vi "BonOMM-SAOMM.vi"() -> ()   [LabVIEW 2019] (continued)
                n727 = local read "XReference"() -> (w1202:dbl)
                n728 = local read "YReference"() -> (w1201:dbl)
                n729 = Greater?(x=w1207, y=w1208) -> (0:w1206:bool)
                n730 = expression code="x/180.0"(3.141592653589793) -> (w1195:dbl)
                n731 = call "xy2ad.vi"("Y (px)"=w1201, "X (px)"=w1202, "Astrometry"=w1203) -> ("DEC (°)"=w1198:dbl, "RA (°)"=w1199:dbl)  [unwired: 5 in, 2 out]
                n732 = call "xy2ad.vi"("Y (px)"=w1204, "X (px)"=w1205, "Astrometry"=w1203) -> ("DEC (°)"=w1196:dbl, "RA (°)"=w1197:dbl)  [unwired: 5 in, 2 out]
                n733 = case shown="Vrai" w1206 {
                  tunnel: w1207 -> [_ w1209]
                  frame False {
                  }
                  frame True {
                    "CorrID" <- w1209
                  }
                }
                n734 = formula code="ErrorRA=(CenRA-RefRA)*3600.0*cos(RefDEC*PIsur180);\nErrorDEC=(CenDEC-RefDEC)*3600.0;"("RefRA"=w1199, "RefDEC"=w1198, "CenRA"=w1197, "CenDEC"=w1196, "PIsur180"=w1195) -> ("ErrorRA"=w1194:dbl, "ErrorDEC"=w1193:dbl)
              }
              frame 2 {
                # "Ajouter une condition sur la dérivée locale ???"
                # "Asservissement Actif (LUT + Servo + Guidage)"
                # "Pas besoin d'appliquer la rotation puisque\nseul l'écart de l'hexapode est considéré."
                n735 = local read "EcartX"() -> (w1219:dbl)
                n736 = local read "EcartY"() -> (w1222:dbl)
                n737 = Absolute Value(x=w1219) -> (abs(x)=w1224:dbl)
                n738 = Absolute Value(x=w1222) -> (abs(x)=w1223:dbl)
                n739 = Greater Or Equal?(x=w1224, y="CorrTreshold") -> (x >= y?=w1218:bool)
                n740 = Less?(x="CorrTreshold", y=w1223) -> (x < y?=w1211:bool)
                n741 = Or(x=w1218, y=w1211) -> (x .or. y?=w1225:bool)
                n742 = Multiply(x=w1219, y="HexXRate") -> (x*y=w1217:dbl)
                n743 = Multiply(x="HexYRate", y=w1222) -> (x*y=w1214:dbl)
                n744 = Select(t=w1214, s=w1211, f=0.0) -> (s? t:f=w1213:dbl)
                n745 = Select(t=w1217, s=w1218, f=0.0) -> (s? t:f=w1215:dbl)
              }
              frame 4 {
                # "On  envoi la commande recu"
                # "Mode Guidage externe"
                n746 = local read "GE_TCS_DEC"() -> (w1232:dbl)
                n747 = local read "GE_TCS_RA"() -> (w1233:dbl)
                n748 = Not Equal To 0?(x=w1232) -> (x != 0?=w1229:bool)
                n749 = local read "GE_TCS"() -> (w1228:bool)
                n750 = Not Equal To 0?(x=w1233) -> (x != 0?=w1230:bool)
                n751 = Or(x=w1230, y=w1229) -> (x .or. y?=w1227:bool)
                n752 = And(x=w1227, y=w1228) -> (x .and. y?=w1231:bool)
                n753 = case shown="Vrai" w1231 {
                  frame False {
                  }
                  frame True {
                    # "On efface la commande"
                    n754 = local read "GE_TCS_DEC"() -> (w1234:dbl)
                    n755 = local read "GE_TCS_RA"() -> (w1240:dbl)
                    n756 = In Range and Coerce(upper limit=5.0, x=w1240, lower limit=-5.0) -> (In Range?=w1243:bool)  [unwired: 1 out]
                    n757 = In Range and Coerce(upper limit=5.0, x=w1234, lower limit=-5.0) -> (In Range?=w1235:bool)  [unwired: 1 out]
                    n758 = case shown="Faux" w1243 {
                      tunnel: w1240 -> [w1252 _]
                      tunnel: [w1253 0.0 ("GE_TCS_RA")] -> w1239
                      frame False {
                        n759 = Greater Than 0?(x=w1252) -> (x > 0?=w1254:bool)
                        n760 = case shown="Faux" w1254 {
                          tunnel: [-5.0 ("y") 5.0 ("y")] -> w1251
                          frame False {
                          }
                          frame True {
                          }
                        }
                        n761 = Subtract(x=w1252, y=w1251) -> (x-y=w1253:dbl)
                      }
                      frame True {
                      }
                    }
                    n762 = case shown="Faux" w1235 {
                      tunnel: [w1247 0.0 ("GE_TCS_DEC")] -> w1238
                      tunnel: w1234 -> [w1246 _]
                      frame False {
                        n763 = Greater Than 0?(x=w1246) -> (x > 0?=w1245:bool)
                        n764 = case shown="Faux" w1245 {
                          tunnel: [-5.0 ("y") 5.0 ("y")] -> w1244
                          frame False {
                          }
                          frame True {
                          }
                        }
                        n765 = Subtract(x=w1246, y=w1244) -> (x-y=w1247:dbl)
                      }
                      frame True {
                      }
                    }
                    n766 = local write "GE_TCS_RA"(w1239) -> ()
                    n767 = local write "GE_TCS_DEC"(w1238) -> ()
                  }
                }
              }
            }
            n768 = Tick Count (ms)() -> (millisecond timer value=w1179:u32)
            n769 = Subtract(x=w1179, y="LastCorr") -> (x-y=w1181:u32)
            n770 = Greater?(x=w1181, y="CorrDelay") -> (0:w1183:bool)
            n771 = local read "SNRtreshold"() -> (w1175:dbl)
            n772 = local read "SNR"() -> (w1176:dbl)
            n773 = local read "Servo"() -> (w1172:bool)
            n774 = Greater Or Equal?(x=w1176, y=w1175) -> (x >= y?=w1173:bool)
            n775 = Compound Arithmetic op=AND(w1173, w1172) -> (w1171:bool)
            n776 = Or(x=w1170, y=w1171) -> (x .or. y?=w1169:bool)
            n777 = Compound Arithmetic op=AND(w1177, w1169, w1183) -> (w1174:bool)
            n778 = case shown="Vrai" w1174 {
              tunnel: w1185 -> [_ w1293]
              tunnel: w1184 -> [_ w1292]
              tunnel: "Corr%" -> [_ w1294]
              frame False {
              }
              frame True {
                w1260 = -5000.0 ("lower limit")
                w1261 = 5000.0 ("x")
                # "millisecond d'activation\ndes relais ..."
                # "À déterminer sur l'ordinateur de BonOMM à OMM\nIl faut refaire le lien quand c'est sur un nouvel ordi"
                n779 = Tick Count (ms)() -> (millisecond timer value=w1296:u32)
                n780 = formula code="EW=(agg/100)*corrX*rRA;\nNS=(agg/100)*corrY*rDEC;"("agg"=w1294, "rRA"="RateRA", "bRA"="BacklashRA", "rDEC"="RateDEC", "bDEC"="BacklashDEC", "corrX"=w1292, "corrY"=w1293) -> ("NS"=w1291:dbl, "EW"=w1290:dbl)
                n781 = local write "LastCorr"(w1296) -> ()
                n782 = local read "path_trackfile"() -> (w1279:path)
                n783 = control-ref of="GuidingCancel"() -> (w1283:refnum<vi>)
                n784 = control-ref of="GuideNorth"() -> (w1284:refnum<vi>)
                n785 = control-ref of="GuideSouth"() -> (w1285:refnum<vi>)
                n786 = control-ref of="GuideEast"() -> (w1282:refnum<vi>)
                n787 = control-ref of="GuideWest"() -> (w1281:refnum<vi>)
                n788 = Round To Nearest(number=w1291) -> (nearest integer value=w1263:dbl)
                n789 = Round To Nearest(number=w1290) -> (nearest integer value=w1262:dbl)
                n790 = Strip Path(path=w1279) -> (stripped path=w1277:path)  [unwired: 1 out]
                n791 = In Range and Coerce(upper limit=w1261, x=w1263, lower limit=w1260) -> (coerced(x)=w1258:dbl)  [unwired: 1 out]
                n792 = In Range and Coerce(upper limit=w1261, x=w1262, lower limit=w1260) -> (coerced(x)=w1259:dbl)  [unwired: 1 out]
                n793 = Bundle("GuidingCancel"=w1283, "GuideNorth"=w1284, "GuideSouth"=w1285, "GuideEast"=w1282, "GuideWest"=w1281) -> (w1280:T27)  [unwired: 1 in]
                n794 = Build Path(base path=w1277, name or relative path="Relays") -> (appended path=w1264:path)
                n795 = local read "RotationTCS"() -> (w1272:dbl)
                n796 = local read "ErrX"() -> (w1270:string)
                n797 = local read "ErrY"() -> (w1269:string)
                n798 = local read "exptime"() -> (w1271:dbl)
                n799 = To Long Integer(number=w1258) -> (32bit integer=w1273:i32)
                n800 = To Long Integer(number=w1259) -> (32bit integer=w1274:i32)
                n801 = Fract/Exp String To Number(string=w1270) -> (number=w1268:dbl)  [unwired: 3 in, 1 out]
                n802 = Fract/Exp String To Number(string=w1269) -> (number=w1267:dbl)  [unwired: 3 in, 1 out]
                n803 = local read "HexX"() -> (w1266:dbl)
                n804 = local read "HexY"() -> (w1265:dbl)
                n805 = call "LogRelayData.vi"("Path"=w1264, "XCorr"=w1273, "YCorr"=w1274, "Rotation"=w1272, "Texp"=w1271, "CenX"=w1268, "CenY"=w1267, "XHex"=w1266, "YHex"=w1265) -> ()  [unwired: 7 in]
                n806 = call "DIO-ApplyCorrection.vi"("TaskCluster"=T21 {"North Task"="Nord", "West Task"="Sud", "South Task"="Est", "East Task"="Ouest"}, "NordSud(ms)"=w1273, "EstOuest(ms)"=w1274, "ReferenceCluster"=w1280) -> ("GuiderRA Error"=w1276:errorcluster, "GuiderDEC Error"=w1275:errorcluster)  [unwired: 10 in]
                n807 = call "LogRelayError.vi"("Path"=w1264, "GuiderRA Error"=w1276, "GuiderDEC Error"=w1275) -> ()  [unwired: 13 in]
              }
            }
            n808 = local read "Quit"() -> (w1178:bool)
            n809 = Wait Until Next ms Multiple(millisecond multiple=u32 50) -> ()  [unwired: 1 out]
          }
          "Guidage" <- w977
          n810 = while {
            tunnel: ["Quit"] -> w982
            stop <- "Quit" stop-if-true
            # "Structure de gestion des événements utilisateurs"
            n811 = event shown="[64] \"BoutonTest\": Valeur changée" {
              selector: _ -> [_ _ _ _ _ _ _ _ _ _ _ _ _ _ _ _ _ _ _ _ _ _ _ _ _ _ _ _ _ _ _ _ _ _ _ _ _ _ _ _ _ _ _ _ _ _ _ _ _ _ _ _ _ _ _ _ _ _ _ _ _ _ _ _ _ _ _ _]
              dyn-events: _ -> [_ _ _ _ _ _ _ _ _ _ _ _ _ _ _ _ _ _ _ _ _ _ _ _ _ _ _ _ _ _ _ _ _ _ _ _ _ _ _ _ _ _ _ _ _ _ _ _ _ _ _ _ _ _ _ _ _ _ _ _ _ _ _ _ _ _ _ _]
              timeout: 250 -> [_ _ _ _ _ _ _ _ _ _ _ _ _ _ _ _ _ _ _ _ _ _ _ _ _ _ _ _ _ _ _ _ _ _ _ _ _ _ _ _ _ _ _ _ _ _ _ _ _ _ _ _ _ _ _ _ _ _ _ _ _ _ _ _ _ _ _ _]
              event Timeout {
                w4204 = FALSE
                # "S'il y a un problème avec MC-BonOMM, regarder ici ;)"
                # "Test pour les boutons de Jog ..."
                n812 = event-data() -> ()  [unwired: 1 in, 1 out]
                n813 = local write "Annulation en cours"(FALSE) -> ()
                n814 = disable-structure shown="Enabled" {
                  frame Disabled {
                    n815 = local read "MC-BonOMM VRN"() -> (w4206:refnum<visa-resource-name>)
                    n816 = property class="Instr"(reference=w4206) -> (reference out=w4207:refnum<visa-resource-name>, "Serial Settings:Number of Bytes at Serial Port"=w4208:u32)  [unwired: 1 in, 1 out]
                    n817 = VISA Read(VISA resource name=w4207, byte count=w4208) -> ()  [unwired: 1 in, 4 out]
                  }
                  frame Enabled {
                  }
                }
                n818 = local write "go Nord"(w4204) -> ()
                n819 = local write "go Ouest"(w4204) -> ()
                n820 = local write "go Est"(w4204) -> ()
                n821 = local write "go Sud"(w4204) -> ()
                n822 = local write "enfoncé"(w4204) -> ()
              }
              event Menu Selection (User) {
                n823 = event-data() -> ("MenuRef"=w4209:refnum<k9>, "ItemTag"=w4211:string, "ItemPath"=w4212:string)  [unwired: 1 in, 3 out]
                n824 = Concatenate Strings(":" ("search string/char (-)"), w4211) -> (w4213:string)
                n825 = Search/Split String(string=w4212, search string/char (-)=w4213) -> (substring before match=w4210:string)  [unwired: 1 in, 2 out]
                n826 = case shown="\"main_Secondaire Actif\"" w4210 {
                  tunnel: w4211 -> [_ w4215 w4532 w4563 w4693 w4768 w4862 w4956 w5019 w5044]
                  tunnel: w4209 -> [_ _ _ _ _ _ w4861 _ _ _]
                  frame Default {
                  }
                  frame "main_Communications" {
                    # "Gestion des éléments du menu \"communications\"\n(fermeture de la connexion, puis redémarrage)"
                    n827 = case shown="\"com_Telescope Control System\"" w4215 {
                      frame Default {
                        (unwired) FALSE ("Boolean")
                      }
                      frame "com_Telescope Control System" {
                        n828 = flat-sequence {
                          frame #0 {
                            w4229 = "communications" ("name or relative path")
                            n829 = control-ref of="TCS actif"() -> (w4218:refnum<vi>)
                            n830 = local read "TCS VRN"() -> (w4223:refnum<visa-resource-name>)
                            n831 = call "EXCOM-25-EQ.vi"("VISA resource name"=w4223, "Bool Refnum"=w4218) -> ("VISA resource name dup"=w4221:refnum<visa-resource-name>, "Error OUT"=w4222:errorcluster)  [unwired: 3 in, 13 out]
                            n832 = local read "properties.ini"() -> (w4225:path)
                            n833 = call "SerialCommError.vi"("VISA IN"=w4221, "error IN"=w4222) -> ("VISA OUT"=w4236:refnum<visa-resource-name>, "Error"=w4224:bool, "error OUT"=w4216:errorcluster)  [unwired: 11 in]
                            n834 = Not(x=w4224) -> (.not. x?=w4217:bool)
                            n835 = call <vilib>:"Open Config Data.vi"("configuration file path"=w4225) -> ("error out"=w4234:errorcluster, "refnum"=w4235:T23)  [unwired: 8 in, 1 out]
                            n836 = local write "TCS VRN"(w4236) -> ()
                            n837 = local write "TCS Error"(w4216) -> ()
                            n838 = case shown="Vrai" w4217 {
                              tunnel: [TRUE ("Boolean") w4279] -> w4219
                              frame False {
                              }
                              frame True {
                                n839 = Two Button Dialog(message="La connexion TCP/IP semble fonctionner.\nDésirez-vous vraiment la réinitialiser ?" ("T button name (\"OK\")"), 1:"Non" ("F button name (\"Cancel\")"), 2:"Oui" ("T button name (\"OK\")")) -> (T button?=w4279:bool)
                              }
                            }
                            n840 = call-poly <vilib>:"Read Key.vi"("section"=w4229, "error in (no error)"=w4234, "key"="TCS-IP" ("name or relative path"), "refnum"=w4235) -> ("error out"=w4232:errorcluster, "value"=w4220:string, "refnum out"=w4233:T23)  [unwired: 4 in, 1 out]
                            n841 = call-poly <vilib>:"Read Key.vi"("section"=w4229, "error in (no error)"=w4232, "key"="TCS-PN" ("name or relative path"), "refnum"=w4233) -> ("error out"=w4230:errorcluster, "value"=w4226:u32, "refnum out"=w4231:T23)  [unwired: 4 in, 1 out]
                            n842 = call <vilib>:"Close Config Data.vi"("error in (no error)"=w4230, "refnum"=w4231) -> ()  [unwired: 8 in, 2 out]
                            n843 = case shown="Vrai" w4219 {
                              tunnel: w4226 -> [_ w4242]
                              tunnel: w4220 -> [_ w4243]
                              tunnel: w4218 -> [_ w4244]
                              frame False {
                              }
                              frame True {
                                n844 = flat-sequence {
                                tunnel: w4244 -> [w4251]
                                tunnel: [refnum<visa-resource-name> "-1" ("Table VRN")] -> w4239
                                tunnel: [w4248] -> w4238
                                tunnel: w4239 -> [w4255]
                                tunnel: w4238 -> [w4254]
                                tunnel: [w4252] -> w4237
                                tunnel: w4237 -> [_]
                                tunnel: w4243 -> [w4262]
                                tunnel: w4242 -> [w4261]
                                tunnel: [w4260] -> w4241
                                tunnel: [w4259] -> w4240
                                tunnel: [w4273] -> w4246
                                tunnel: [w4272] -> w4245
                                tunnel: w4240 -> [_]
                                tunnel: w4241 -> [w4267]
                                tunnel: w4246 -> [w4275]
                                tunnel: w4245 -> [w4274]
                                frame #0 {
                                w4247 = TRUE ("TCS R actif")
                                n845 = local write "ReconnectionMute"(w4247) -> ()
                                n846 = local read "TCS VRN"() -> (w4248:refnum<visa-resource-name>)
                                n847 = call "TCS-Wait4Flag.vi"("Raise Flag ?"=TRUE, "Ctl Refnum IN"=w4251) -> ()  [unwired: 8 in, 2 out]
                                "TCSMute" <- w4247
                                }
                                frame #1 {
                                n848 = local write "TCS VRN"(w4255) -> ()
                                n849 = Type Cast(type=refnum<k5> refnum ("connection ID out"), x=w4254) -> (*(type *) &x=w4256:refnum<k5>)
                                n850 = TCP Close Connection(connection ID=w4256) -> (error out=w4252:errorcluster)  [unwired: 2 in, 1 out]
                                }
                                frame #2 {
                                n851 = Wait (ms)(milliseconds to wait=u32 1000) -> ()  [unwired: 1 out]
                                }
                                frame #3 {
                                n852 = To Unsigned Word Integer(number=w4261) -> (unsigned 16bit integer=w4263:u16)
                                n853 = local write "TCS actif"(FALSE ("TCS R actif")) -> ()
                                n854 = TCP Open Connection(address=w4262, remote port or service name=w4263) -> (connection ID=w4260:refnum<k5>, error out=w4259:errorcluster)  [unwired: 3 in]
                                }
                                frame #4 {
                                # "Doit-on fermer la \nconnexion d'abord ?"
                                n855 = Type Cast(type="", x=w4267) -> (*(type *) &x=w4270:string)
                                n856 = control-ref of="TCS actif"() -> (w4264:refnum<vi>)
                                n857 = Type Cast(type=refnum<visa-resource-name> "-1" ("Table VRN"), x=w4270) -> (*(type *) &x=w4268:refnum<visa-resource-name>)
                                n858 = call "EXCOM-25-EQ.vi"("VISA resource name"=w4268, "Bool Refnum"=w4264) -> ("VISA resource name dup"=w4266:refnum<visa-resource-name>, "Error OUT"=w4265:errorcluster)  [unwired: 3 in, 13 out]
                                n859 = call "SerialCommError.vi"("VISA IN"=w4266, "error IN"=w4265) -> ("VISA OUT"=w4273:refnum<visa-resource-name>, "error OUT"=w4272:errorcluster)  [unwired: 11 in, 1 out]
                                }
                                frame #5 {
                                n860 = case shown="Erreur" w4274 {
                                frame No Error {
                                }
                                frame Error {
                                n861 = One Button Dialog(message="La communication avec le TCS ne semble toujours pas foncitonner.\nVérifiez les connexions et les paramètres puis recommencez." ("T button name (\"OK\")")) -> ()  [unwired: 1 in, 1 out]
                                }
                                }
                                n862 = local write "TCS Error"(w4274) -> ()
                                n863 = local write "TCS VRN"(w4275) -> ()
                                }
                                frame #6 {
                                w4277 = FALSE
                                n864 = local write "ReconnectionMute"(w4277) -> ()
                                n865 = local write "TCSMute"(w4277) -> ()
                                }
                                }
                              }
                            }
                          }
                        }
                      }
                      frame "com_Caméra de référence" {
                        n866 = local read "exptime"() -> (w4285:dbl)
                        n867 = local read "MessageType"() -> (w4290:cluster{string[], u32[]})
                        n868 = control-ref of="PrAMS-ACK"() -> (w4295:refnum<vi>)
                        n869 = control-ref of="PrAMS actif"() -> (w4294:refnum<vi>)
                        n870 = local read "Signature"() -> (w4293:u32)
                        n871 = local read "PrAMS VRN"() -> (w4296:refnum<visa-resource-name>)
                        n872 = expression code="x*1000"(w4285) -> (w4288:dbl)
                        n873 = To Unsigned Long Integer(number=w4288) -> (unsigned 32bit integer=w4287:u32)
                        n874 = call-poly "SAOMM-Num2littleEndian.vi"("Number"=w4287) -> ("LiitleEndianedData"=w4286:u8[])  [unwired: 14 in]
                        n875 = call "SAOMM-SendSET.vi"("PRAMMS-COMM IN"=w4296, "Active Refnum"=w4294, "PrAMS-ACK"=w4295, "Signature"=w4293, "Error IN"=errorcluster {"status"=FALSE, "code"=0, "source"=""} ("PRAMMS Error"), "MessageType"=w4290, "Active SET"="emtSetImageExposureTime", "Value (little endianed byte array)"=w4286) -> ("Error"=w4284:bool, "Error OUT"=w4292:errorcluster)  [unwired: 4 in, 2 out]
                        n876 = local write "PrAMS Error"(w4292) -> ()
                        n877 = Not(x=w4284) -> (.not. x?=w4283:bool)
                        n878 = case shown="Vrai" w4283 {
                          tunnel: [TRUE ("Boolean") w4299] -> w4297
                          frame False {
                          }
                          frame True {
                            n879 = Two Button Dialog(message="La connexion TCP/IP semble fonctionner.\nDésirez-vous vraiment la réinitialiser ?" ("T button name (\"OK\")"), 1:"Non" ("F button name (\"Cancel\")"), 2:"Oui" ("T button name (\"OK\")")) -> (T button?=w4299:bool)
                          }
                        }
                        n880 = case shown="Vrai" w4297 {
                          frame False {
                          }
                          frame True {
                            n881 = flat-sequence {
                              tunnel: [w4304] -> w4303
                              tunnel: w4303 -> [_]
                              frame #0 {
                                n882 = local read "PrAMS VRN"() -> (w4306:refnum<visa-resource-name>)
                                n883 = Type Cast(type=refnum<k5> refnum ("connection ID"), x=w4306) -> (*(type *) &x=w4305:refnum<k5>)
                                n884 = TCP Close Connection(connection ID=w4305) -> (error out=w4304:errorcluster)  [unwired: 2 in, 1 out]
                              }
                              frame #1 {
                                n885 = local read "properties.ini"() -> (w4316:path)
                                n886 = local read "path_config"() -> (w4309:path)
                                n887 = Build Path(base path=w4309, name or relative path=path "command.ini" ("command.ini")) -> (appended path=w4308:path)
                                n888 = call <vilib>:"Open Config Data.vi"("create file if necessary (T)"=FALSE, "configuration file path"=w4316) -> ("error out"=w4314:errorcluster, "refnum"=w4313:T23)  [unwired: 7 in, 1 out]
                                n889 = local read "Signature"() -> (w4325:u32)
                                n890 = call-poly <vilib>:"Read Key.vi"("section"="communications" ("key"), "error in (no error)"=w4314, "key"="PRAMMS-IP", "refnum"=w4313) -> ("error out"=w4320:errorcluster, "value"=w4312:string, "refnum out"=w4319:T23)  [unwired: 4 in, 1 out]
                                n891 = call <vilib>:"Close Config Data.vi"("error in (no error)"=w4320, "refnum"=w4319) -> ()  [unwired: 8 in, 2 out]
                                n892 = call "SAOMM-connect.vi"("IP"=w4312, "Port"=u16 10010, "Signature"=w4325, "Command.ini"=w4308) -> ("connection ID"=w4322:refnum<k5>, "Error OUT"=w4311:errorcluster)  [unwired: 7 in, 3 out]
                                n893 = disable-structure shown="Disabled" {
                                disable-tunnel: w4311 -> [w4327 _]
                                frame Disabled {
                                n894 = case shown="Erreur" w4327 {
                                frame No Error {
                                }
                                frame Error {
                                n895 = One Button Dialog(message="Erreur lors de la connexion\nà l'hexapode-console.") -> ()  [unwired: 1 in, 1 out]
                                }
                                }
                                }
                                frame Enabled {
                                }
                                }
                                n896 = local read "PrAMS VRN"() -> (w4324:refnum<visa-resource-name>)
                                n897 = local write "PrAMS Error"(w4311) -> ()
                                n898 = Type Cast(type=w4312, x=w4322) -> (*(type *) &x=w4321:string)
                                n899 = Type Cast(type=w4324, x=w4321) -> (*(type *) &x=w4323:refnum<visa-resource-name>)
                                n900 = local write "PrAMS VRN"(w4323) -> ()
                              }
                            }
                          }
                        }
                      }
                      frame "com_Tables de guidage" {
                        n901 = flat-sequence {
                          frame #0 {
                            w4330 = TRUE
                            n902 = local write "Sync_Ready"(FALSE ("Sync_Ready")) -> ()
                            "TableMute" <- w4330
                            "ReconnectionMute" <- w4330
                          }
                          frame #1 {
                            w4345 = "communications" ("name or relative path")
                            n903 = local read "Table VRN"() -> (w4334:refnum<visa-resource-name>)
                            n904 = local read "properties.ini"() -> (w4338:path)
                            n905 = control-ref of="Table actif"() -> (w4332:refnum<vi>)
                            n906 = local read "ActiveStages"() -> (w4331:string[])
                            n907 = call "Newmark-Status-All.vi"("Table VRN IN"=w4334, "Bool Refnum"=w4332, "StageTag"=w4331) -> ("Table VRN OUT"=w4335:refnum<visa-resource-name>, "Error OUT"=w4333:errorcluster)  [unwired: 4 in, 11 out]
                            n908 = call <vilib>:"Open Config Data.vi"("configuration file path"=w4338) -> ("error out"=w4350:errorcluster, "refnum"=w4351:T23)  [unwired: 8 in, 1 out]
                            n909 = call "SerialCommError.vi"("VISA IN"=w4335, "error IN"=w4333) -> ("VISA OUT"=w4352:refnum<visa-resource-name>, "Error"=w4336:bool)  [unwired: 11 in, 1 out]
                            n910 = case shown="Vrai" w4336 {
                              selector: w4336 -> [_ w4365]
                              tunnel: [w4361 w4365] -> w4337
                              frame False {
                                n911 = Two Button Dialog(message="La communication avec les tables semble bonne.\nDésirez-vous vraiment le réinitialiser ?" ("T button name (\"OK\")"), 1:"Non" ("F button name (\"Cancel\")"), 2:"Oui" ("T button name (\"OK\")")) -> (T button?=w4361:bool)
                              }
                              frame True {
                              }
                            }
                            n912 = call-poly <vilib>:"Read Key.vi"("section"=w4345, "error in (no error)"=w4350, "key"="tablevrn" ("name or relative path"), "refnum"=w4351) -> ("error out"=w4348:errorcluster, "value"=w4341:string, "refnum out"=w4349:T23)  [unwired: 4 in, 1 out]
                            n913 = local write "Table VRN"(w4352) -> ()
                            n914 = call-poly <vilib>:"Read Key.vi"("section"=w4345, "error in (no error)"=w4348, "key"="tablespd" ("name or relative path"), "refnum"=w4349) -> ("error out"=w4346:errorcluster, "value"=w4342:u32, "refnum out"=w4347:T23)  [unwired: 4 in, 1 out]
                            n915 = Type Cast(type=refnum<visa-resource-name> "-1" ("TCS R VRN"), x=w4341) -> (*(type *) &x=w4339:refnum<visa-resource-name>)
                            n916 = call <vilib>:"Close Config Data.vi"("error in (no error)"=w4346, "refnum"=w4347) -> ()  [unwired: 8 in, 2 out]
                            n917 = case shown="Vrai" w4337 {
                              tunnel: w4342 -> [_ w4358]
                              tunnel: w4339 -> [_ w4357]
                              frame False {
                              }
                              frame True {
                                n918 = local write "Table Baud rate"(w4358) -> ()
                                n919 = control-ref of="Table actif"() -> (w4355:refnum<vi>)
                                n920 = local read "ActiveStages"() -> (w4356:string[])
                                n921 = call "Newmark-Initialize.vi"("VISA resource name"=w4357, "ActiveStages"=w4356, "baud rate"=w4358, "Timeout"=u32 1000, "Bool Refnum"=w4355) -> ("VISA resource name out"=w4359:refnum<visa-resource-name>, "Error OUT"=w4353:errorcluster)  [unwired: 8 in, 1 out]
                                n922 = local write "Table Error"(w4353) -> ()
                                n923 = case shown="Pas d'erreur" w4353 {
                                frame No Error {
                                }
                                frame Error {
                                n924 = One Button Dialog(message="La communication avec les tables  ne semble toujours pas foncitonner.\nVérifiez les connexions et les paramètres puis recommencez." ("T button name (\"OK\")")) -> ()  [unwired: 1 in, 1 out]
                                }
                                }
                                n925 = local write "Table VRN"(w4359) -> ()
                              }
                            }
                          }
                          frame #2 {
                            w4367 = FALSE
                            n926 = local write "ReconnectionMute"(w4367) -> ()
                            n927 = local write "Sync_Ready"(TRUE ("Sync_Ready")) -> ()
                            n928 = local write "TableMute"(w4367) -> ()
                          }
                        }
                      }
                      frame "com_Secondaire Actif" {
                        (unwired) FALSE
                        w4377 = "communications" ("name or relative path")
                        n929 = local read "properties.ini"() -> (w4372:path)
                        n930 = call <vilib>:"Open Config Data.vi"("configuration file path"=w4372) -> ("error out"=w4382:errorcluster, "refnum"=w4383:T23)  [unwired: 8 in, 1 out]
                        n931 = One Button Dialog(message="À compléter ...") -> ()  [unwired: 1 in, 1 out]
                        n932 = call-poly <vilib>:"Read Key.vi"("section"=w4377, "error in (no error)"=w4382, "key"="PRAMMS-IP" ("name or relative path"), "refnum"=w4383) -> ("error out"=w4380:errorcluster, "value"=w4374:string, "refnum out"=w4381:T23)  [unwired: 4 in, 1 out]
                        n933 = call-poly <vilib>:"Read Key.vi"("section"=w4377, "error in (no error)"=w4380, "key"="PRAMMS-IP" ("name or relative path"), "refnum"=w4381) -> ("error out"=w4378:errorcluster, "value"=w4371:u32, "refnum out"=w4379:T23)  [unwired: 4 in, 1 out]
                        n934 = Type Cast(type=refnum<visa-resource-name> "-1" ("TCS R VRN"), x=w4374) -> (*(type *) &x=w4370:refnum<visa-resource-name>)
                        n935 = call <vilib>:"Close Config Data.vi"("error in (no error)"=w4378, "refnum"=w4379) -> ()  [unwired: 8 in, 2 out]
                        n936 = case shown="Vrai" TRUE {
                          tunnel: w4371 -> [_ _]
                          tunnel: w4370 -> [_ _]
                          frame False {
                          }
                          frame True {
                          }
                        }
                      }
                      frame "com_Lampes de calibration" {
                        n937 = flat-sequence {
                          frame #0 {
                            w4391 = "communications" ("name or relative path")
                            n938 = local read "properties.ini"() -> (w4384:path)
                            n939 = call <vilib>:"Open Config Data.vi"("configuration file path"=w4384) -> ("error out"=w4386:errorcluster, "refnum"=w4385:T23)  [unwired: 8 in, 1 out]
                            n940 = call-poly <vilib>:"Read Key.vi"("section"=w4391, "error in (no error)"=w4386, "key"="calibvrn" ("name or relative path"), "refnum"=w4385) -> ("error out"=w4388:errorcluster, "value"=w4394:string, "refnum out"=w4387:T23)  [unwired: 4 in, 1 out]
                            n941 = call-poly <vilib>:"Read Key.vi"("section"=w4391, "error in (no error)"=w4388, "key"="calibspd" ("name or relative path"), "refnum"=w4387) -> ("error out"=w4390:errorcluster, "value"=w4397:u32, "refnum out"=w4389:T23)  [unwired: 4 in, 1 out]
                            n942 = Type Cast(type=refnum<visa-resource-name> "-1" ("TCS R VRN"), x=w4394) -> (*(type *) &x=w4396:refnum<visa-resource-name>)
                            n943 = call <vilib>:"Close Config Data.vi"("error in (no error)"=w4390, "refnum"=w4389) -> ()  [unwired: 8 in, 2 out]
                            n944 = call-poly "VISA Configure Serial Port"("VISA resource name"=w4396, "timeout (10sec)"=u32 2000, "Enable Termination\nChar (T)"=FALSE ("Enable Termination\nChar (T)"), "baud rate (9600)"=w4397) -> ("VISA resource name out"=w4400:refnum<visa-resource-name>, "error out"=w4401:errorcluster)  [unwired: 10 in]
                            n945 = call "SerialCommError.vi"("VISA IN"=w4400, "error IN"=w4401) -> ("VISA OUT"=w4402:refnum<visa-resource-name>)  [unwired: 11 in, 2 out]
                            n946 = local write "Calib VRN"(w4402) -> ()
                          }
                          frame #1 {
                            n947 = One Button Dialog(message="Le port série des lampes de calibration a été réinitialisé.\n(Aucun test réel car la communication est à sens unique)") -> ()  [unwired: 1 in, 1 out]
                          }
                        }
                      }
                      frame "com_Commandes externes" {
                        (unwired) TRUE
                        n948 = flat-sequence {
                          frame #0 {
                            w4412 = "communications" ("name or relative path")
                            n949 = local read "properties.ini"() -> (w4405:path)
                            n950 = call <vilib>:"Open Config Data.vi"("configuration file path"=w4405) -> ("error out"=w4407:errorcluster, "refnum"=w4406:T23)  [unwired: 8 in, 1 out]
                            n951 = call-poly <vilib>:"Read Key.vi"("section"=w4412, "error in (no error)"=w4407, "key"="excvrn" ("name or relative path"), "refnum"=w4406) -> ("error out"=w4409:errorcluster, "value"=w4415:string, "refnum out"=w4408:T23)  [unwired: 4 in, 1 out]
                            n952 = call-poly <vilib>:"Read Key.vi"("section"=w4412, "error in (no error)"=w4409, "key"="excspd" ("name or relative path"), "refnum"=w4408) -> ("error out"=w4411:errorcluster, "value"=w4418:u32, "refnum out"=w4410:T23)  [unwired: 4 in, 1 out]
                            n953 = Type Cast(type=refnum<visa-resource-name> "-1" ("TCS R VRN"), x=w4415) -> (*(type *) &x=w4417:refnum<visa-resource-name>)
                            n954 = call <vilib>:"Close Config Data.vi"("error in (no error)"=w4411, "refnum"=w4410) -> ()  [unwired: 8 in, 2 out]
                            n955 = call-poly "VISA Configure Serial Port"("VISA resource name"=w4417, "timeout (10sec)"=u32 2000, "Enable Termination\nChar (T)"=FALSE ("Enable Termination\nChar (T)"), "baud rate (9600)"=w4418) -> ("VISA resource name out"=w4421:refnum<visa-resource-name>, "error out"=w4422:errorcluster)  [unwired: 10 in]
                            n956 = call "SerialCommError.vi"("VISA IN"=w4421, "error IN"=w4422) -> ("VISA OUT"=w4404:refnum<visa-resource-name>)  [unwired: 11 in, 2 out]
                            n957 = local write "Excmd VRN"(w4404) -> ()
                          }
                          frame #1 {
                            n958 = One Button Dialog(message="Le port série des communications externes a été réinitialisé.\n(Relancez une commande externe afin de tester la communication)") -> ()  [unwired: 1 in, 1 out]
                          }
                        }
                      }
                      frame "com_MC-BonOMM" {
                        n959 = local read "Périphérique"() -> (w4433:u16)
                        n960 = Two Button Dialog(message="Ceci va redémarrer le contrôleur de roue à filtre\net réinitialiser la communication.\nVoulez-vous continuer ?", 1:"NON" ("F button name (\"Cancel\")"), 2:"OUI" ("T button name (\"OK\")")) -> (T button?=w4424:bool)
                        n961 = Equal?(x=w4433, y=u16 0) -> (x = y?=w4435:bool)
                        n962 = Equal?(x=w4433, y=u16 1) -> (x = y?=w4434:bool)
                        n963 = Equal?(x=w4433, y=u16 2) -> (x = y?=w4436:bool)
                        n964 = Build Array(w4435, w4434, w4436) -> (w4428:bool[])
                        n965 = Boolean Array To Number(Boolean array=w4428) -> (number=w4429:u32)
                        n966 = case shown="Vrai" w4424 {
                          tunnel: w4429 -> [_ w4440]
                          tunnel: [w4437 w4438] -> _
                          frame False {
                            n967 = local read "MC_connect"() -> (w4437:bool)
                          }
                          frame True {
                            n968 = flat-sequence {
                              tunnel: w4440 -> [w4444]
                              tunnel: [w4444] -> w4439
                              tunnel: w4439 -> [w4464]
                              tunnel: [w4450] -> w4438
                              frame #0 {
                                n969 = local read "MC-BonOMM VRN"() -> (w4443:refnum<visa-resource-name>)
                                n970 = flat-sequence {
                                tunnel: w4441 -> [w4448]
                                frame #0 {
                                n971 = Wait (ms)(milliseconds to wait=u32 2000) -> ()  [unwired: 1 out]
                                }
                                frame #1 {
                                n972 = property class="Instr"(reference=w4448) -> (reference out=w4447:refnum<visa-resource-name>, "Serial Settings:Number of Bytes at Serial Port"=w4446:u32)  [unwired: 1 in, 1 out]
                                n973 = local write "MC_connect"(FALSE ("MC_connect")) -> ()
                                n974 = VISA Read(VISA resource name=w4447, byte count=w4446) -> ()  [unwired: 1 in, 4 out]
                                }
                                }
                                n975 = VISA Write(VISA resource name=w4443, write buffer="r" ("Commande")) -> (VISA resource name out=w4441:refnum<visa-resource-name>)  [unwired: 1 in, 2 out]
                              }
                              frame #1 {
                                n976 = local read "MC-BonOMM VRN"() -> (w4460:refnum<visa-resource-name>)
                                n977 = call "MC-BonOMM_talker.vi"("MC-BonOMM VRN"=w4460, "Commande"="m", "byte count"=u32 1, "Timeout (ms)"=2000, "answer=command?"=FALSE) -> ("Answer"=w4454:string, "ok ?"=w4457:bool)
                                n978 = Equal?(x="f", y=w4454) -> (x = y?=w4453:bool)
                                n979 = Equal?(x=w4454, y="x") -> (x = y?=w4452:bool)
                                n980 = Or(x=w4453, y=w4452) -> (x .or. y?=w4451:bool)
                                n981 = And(x=w4451, y=w4457) -> (x .and. y?=w4458:bool)
                                n982 = case shown="Vrai" w4458 {
                                tunnel: w4464 -> [_ w4470]
                                tunnel: [w4465 w4469] -> w4450
                                frame False {
                                n983 = One Button Dialog(message="Problème de communication avec MC-BonOMM", button name ("OK")="Oups :(") -> (true=w4466:bool)
                                n984 = Not(x=w4466) -> (.not. x?=w4465:bool)
                                }
                                frame True {
                                n985 = stacked-sequence {
                                tunnel: w4470 -> [w4472 w4483]
                                tunnel: [_ w4481] -> w4469
                                frame #0 {
                                n986 = case shown="1, Par défaut" w4472 {
                                tunnel: ["f" "o" "x"] -> w4471
                                frame 1, Default {
                                }
                                frame 2 {
                                }
                                frame 4 {
                                }
                                }
                                n987 = local read "MC-BonOMM VRN"() -> (w4475:refnum<visa-resource-name>)
                                n988 = call "MC-BonOMM_talker.vi"("MC-BonOMM VRN"=w4475, "Commande"=w4471, "Timeout (ms)"=2000, "answer=command?"=TRUE) -> ("ok ?"=w4473:bool)  [unwired: 1 in, 1 out]
                                n989 = case shown="Faux" w4473 {
                                frame False {
                                n990 = One Button Dialog(message="Erreur lors du changement de mode ...") -> ()  [unwired: 1 in, 1 out]
                                }
                                frame True {
                                }
                                }
                                n991 = local write "MC_connect"(w4473) -> ()
                                }
                                frame #1 {
                                n992 = local read "MC-BonOMM VRN"() -> (w4482:refnum<visa-resource-name>)
                                n993 = case shown="1, 2, Par défaut" w4483 {
                                tunnel: w4482 -> [w4489 w4499]
                                tunnel: [w4487 w4498] -> w4481
                                frame 1, 2, Default {
                                n994 = call "MC-BonOMM_talker.vi"("MC-BonOMM VRN"=w4489, "Commande"="q", "byte count"=u32 1, "Timeout (ms)"=8000, "answer=command?"=FALSE) -> ("Answer"=w4488:string, "ok ?"=w4487:bool)
                                n995 = Decimal String To Number(string=w4488) -> (number=w4492:i32)  [unwired: 2 in, 1 out]
                                n996 = local write "F#"(w4492) -> ()
                                n997 = case shown="1..6" w4492 {
                                selector: w4492 -> [w4494 _]
                                tunnel: [w4493 ""] -> w4491
                                frame 1..6 {
                                n998 = local read "Tableau des filtres"() -> (w4495:string[])
                                n999 = Decrement(x=w4494) -> (x-1=w4496:i32)
                                n1000 = Index Array(array=w4495, index=w4496) -> (element=w4493:string)
                                }
                                frame 0, Default {
                                }
                                }
                                n1001 = local write "filtre_nom"(w4491) -> ()
                                }
                                frame 4 {
                                n1002 = local read "ST_SPD"() -> (w4500:dbl)
                                n1003 = call "Change_speed.vi"("ST_SPD"=w4500, "MC-BonOMM VRN"=w4499) -> ("Connected?"=w4498:bool)
                                n1004 = case shown="Faux" w4498 {
                                frame False {
                                n1005 = property on="Périphérique" class="MDér (strict)"("Value (Signaling)"=u16 3) -> ()  [unwired: 2 in, 2 out]
                                }
                                frame True {
                                }
                                }
                                }
                                }
                                }
                                }
                                }
                                }
                                n1006 = local write "MC_connect"(w4450) -> ()
                              }
                            }
                          }
                        }
                      }
                      frame "com_Station Météo" {
                        # "Réinitialisation de la connexion avec le cRIO de météo"
                        n1007 = flat-sequence {
                          tunnel: [w4508] -> w4503
                          tunnel: w4503 -> [w4526]
                          tunnel: [w4526] -> w4502
                          frame #0 {
                            # "Ferme la connexion si elle est ouverte"
                            n1008 = local read "Cx"() -> (w4504:bool)
                            n1009 = case shown="Vrai" w4504 {
                              frame False {
                              }
                              frame True {
                                n1010 = local read "cRIO_commID"() -> (w4505:refnum<k5>)
                                n1011 = TCP Close Connection(connection ID=w4505) -> ()  [unwired: 2 in, 2 out]
                              }
                            }
                          }
                          frame #1 {
                            n1012 = local read "cRIO Port"() -> (w4506:u16)
                            n1013 = local read "cRIO address"() -> (w4512:string)
                            n1014 = TCP Open Connection(address=w4512, remote port or service name=w4506) -> (connection ID=w4513:refnum<k5>, error out=w4510:errorcluster)  [unwired: 3 in]
                            n1015 = Unbundle By Name(w4510) -> ("status"=w4511:bool)
                            n1016 = local write "cRIO_commID"(w4513) -> ()
                            n1017 = Not(x=w4511) -> (.not. x?=w4507:bool)
                            n1018 = local write "Cx"(w4507) -> ()
                            n1019 = case shown="Vrai" w4507 {
                              tunnel: [errorcluster {"status"=FALSE, "code"=0, "source"=""} ("error out") w4516] -> w4509
                              frame False {
                                w4515 = 0.0 ("indic-T-out")
                                n1020 = local write "indic-Tm"(w4515) -> ()
                                n1021 = local write "indic-T-struct"(w4515) -> ()
                                n1022 = local write "indic-T-out"(w4515) -> ()
                                n1023 = local write "indic-T-in"(w4515) -> ()
                                n1024 = local write "indic-H-out"(w4515) -> ()
                                n1025 = local write "indic-H-in"(w4515) -> ()
                              }
                              frame True {
                                n1026 = local read "cRIO_commID"() -> (w4524:refnum<k5>)
                                n1027 = call "TCP-read.vi"("connection ID"=w4524) -> ("error out"=w4516:errorcluster, "data out"=w4525:string)  [unwired: 2 in, 1 out]
                                n1028 = call "line2array.vi"("data-line"=w4525) -> ("data-array"=w4523:dbl[])  [unwired: 2 out]
                                n1029 = Index Array(array=w4523) -> (element #1=w4522:dbl, element #2=w4521:dbl, element #3=w4520:dbl, element #4=w4519:dbl, element #7=w4518:dbl, element #8=w4517:dbl)  [unwired: 9 in, 3 out]
                                n1030 = local write "indic-Tm"(w4518) -> ()
                                n1031 = local write "indic-T-struct"(w4517) -> ()
                                n1032 = local write "indic-T-out"(w4522) -> ()
                                n1033 = local write "indic-T-in"(w4520) -> ()
                                n1034 = local write "indic-H-out"(w4521) -> ()
                                n1035 = local write "indic-H-in"(w4519) -> ()
                              }
                            }
                            n1036 = Unbundle By Name(w4509) -> ("status"=w4508:bool)
                          }
                          frame #2 {
                            n1037 = case shown="Vrai" w4526 {
                              frame False {
                              }
                              frame True {
                                n1038 = One Button Dialog(message="La communication avec la station météo n'a pu être rétablie.\nVérifier les connexions réseaux ou redémarrer le système.") -> ()  [unwired: 1 in, 1 out]
                              }
                            }
                          }
                        }
                        n1039 = Not(x=w4502) -> ()  [unwired: 1 out]
                      }
                      frame "com_Caméra de guidage" {
                        (unwired) FALSE ("Boolean")
                      }
                      frame "com_Reconnexion automatique ?" {
                        n1040 = local read "AutoConnect?"() -> (w4529:bool)
                        n1041 = Not(x=w4529) -> (.not. x?=→"AutoConnect?":bool)
                      }
                    }
                  }
                  frame "main_Instruments" {
                    # "Ajouter le charement de la LUT approprié ..."
                    n1042 = String Subset(string=w4532, offset (0)=4) -> (substring=w4531:string)  [unwired: 1 in]
                    n1043 = local read "Instrument Actuel"() -> (w4533:string)
                    n1044 = Not Equal?(x=w4531, y=w4533) -> (x != y?=w4534:bool)
                    n1045 = case shown="Vrai" w4534 {
                      tunnel: w4531 -> [_ w4549]
                      tunnel: w4533 -> [_ w4545]
                      frame False {
                      }
                      frame True {
                        n1046 = local read "instruments.ini"() -> (w4550:path)
                        n1047 = Current VI's Menubar() -> (w4548:refnum<k9>)
                        n1048 = Set Menu Item Info(6:FALSE ("checked"), 7:w4545, 11:w4548) -> (0:w4546:errorcluster, 3:w4547:refnum<k9>)  [unwired: 4 in]
                        n1049 = call "InstrChoice.vi"("Instrument IN"=w4549, "instruments.ini"=w4550, "DisallowUndo"=FALSE) -> ("Modifier?"=w4535:bool, "Instrument OUT"=w4542:string, "FoV"=w4540:dbl, "foynom"=w4541:i32, "atherm"=w4539:dbl, "exclusion"=w4538:path, "collim"=w4537:path)  [unwired: 9 in, 1 out]
                        n1050 = Set Menu Item Info(6:TRUE ("checked"), 7:w4542, 8:w4546, 11:w4547) -> ()  [unwired: 3 in, 2 out]
                        n1051 = case shown="Vrai" w4535 {
                          tunnel: w4542 -> [_ w4562]
                          tunnel: w4541 -> [_ w4561]
                          tunnel: w4540 -> [_ w4560]
                          tunnel: w4539 -> [_ w4559]
                          tunnel: w4538 -> [_ w4558]
                          tunnel: w4537 -> [_ w4552]
                          frame False {
                          }
                          frame True {
                            n1052 = local write "Instrument Actuel"(w4562) -> ()
                            n1053 = local write "path_exclusion"(w4558) -> ()
                            n1054 = local write "FOV"(w4560) -> ()
                            n1055 = local write "Foyer à 0°"(w4561) -> ()
                            n1056 = local write "Ath_coef"(w4559) -> ()
                            n1057 = local write "ActiveLUT"(w4552) -> ()
                            n1058 = call "SAOMM-XML2LUT.vi"("Path"=w4552) -> ("NominalPositions"=w4551:dbl[])  [unwired: 13 in, 1 out]
                            n1059 = Index Array(array=w4551) -> (element #3=w4557:dbl, element #4=w4556:dbl, element #5=w4555:dbl, element #6=w4554:dbl, element #7=w4553:dbl)  [unwired: 7 in, 2 out]
                            n1060 = local write "Nominal Y"(w4556) -> ()
                            n1061 = local write "Nominal X"(w4557) -> ()
                            n1062 = local write "Nominal Z"(w4555) -> ()
                            n1063 = local write "Nominal V"(w4553) -> ()
                            n1064 = local write "Nominal U"(w4554) -> ()
                          }
                        }
                      }
                    }
                  }
                  frame "main_Scripts et Automatismes" {
                    n1065 = case shown="\"scp_Charger la librairie Pesto\"" w4563 {
                      selector: w4563 -> [w4567 _ _ _ _ _ _]
                      frame "", Default {
                        n1066 = Concatenate Strings("Erreur avec le menu, cela ne devrait pas se produire ...\nCommande : (\"" ("message"), w4567, "\")" ("message")) -> (w4565:string)
                        n1067 = One Button Dialog(message=w4565) -> ()  [unwired: 1 in, 1 out]
                      }
                      frame "scp_Charger la librairie CPAPIR" {
                        n1068 = local read "properties.ini"() -> (w4568:path)
                        n1069 = local read "path_libdir"() -> (w4571:path)
                        n1070 = call "Get_properties.vi"("Keyword"="queuelib" ("Section"), "Section"="chemins", "properties.ini"=w4568) -> ("error"=w4572:bool, "string"=w4570:string)  [unwired: 6 in, 1 out]
                        n1071 = case shown="Faux" w4572 {
                          tunnel: w4571 -> [w4578 _]
                          tunnel: w4570 -> [w4587 _]
                          tunnel: "table_technicien.dat" -> [w4584 _]
                          frame False {
                            n1072 = Build Path(base path=w4578, name or relative path=w4584) -> (appended path=w4583:path)
                            n1073 = File/Directory Info(path=w4583) -> (path out=w4580:path, error out=w4582:errorcluster)  [unwired: 1 in, 5 out]
                            n1074 = Unbundle By Name(w4582) -> ("status"=w4581:bool)
                            n1075 = local read "wgetexec"() -> (w4585:path)
                            n1076 = case shown="Faux" w4581 {
                              tunnel: w4580 -> [w4610 w4612]
                              tunnel: [w4609 w4612] -> w4579
                              tunnel: w4578 -> [w4608 w4611]
                              tunnel: [w4608 w4611] -> w4577
                              frame False {
                                n1077 = Delete(path (use dialog)=w4610) -> (deleted path=w4609:path)  [unwired: 4 in, 2 out]
                              }
                              frame True {
                              }
                            }
                            n1078 = Path To String(path=w4585) -> (string=w4575:string)
                            n1079 = Concatenate Strings(w4575, " --http-user=carpe", " --http-password=noctem ", w4587) -> (w4590:string)
                            n1080 = call <vilib>:"System Exec.vi"("run minimized? (F)"=TRUE, "working directory"=w4577, "command line"=w4590) -> ("error out"=w4576:errorcluster)  [unwired: 5 in, 3 out]
                            n1081 = flat-sequence {
                              tunnel: w4579 -> [w4594]
                              tunnel: w4576 -> [w4591]
                              frame #0 {
                                n1082 = local write "wget error"(w4591) -> ()
                                n1083 = call "Read_obs_files.vi"("Path"=w4594) -> ("path used"=w4592:path, "Output Table"=w4596:string[][])
                                n1084 = local read "LST"() -> (w4595:dbl)
                                n1085 = for {
                                tunnel: w4596 -> [w4602] mode=indexing
                                tunnel: w4595 -> [w4603]
                                tunnel: [w4599] -> w4593 mode=indexing
                                n1086 = Index Array(array=w4602, index #1=2 ("index"), index #2=3 ("index")) -> (element #1=w4605:string, element #2=w4604:string)
                                n1087 = call "Airmass.vi"("temps sidéral"=w4603, "DEC"=w4604, "RA"=w4605) -> ("airmass"=w4600:dbl)
                                n1088 = Number To Fractional String(number=w4600, precision (6)=i16 2) -> (F-format string=w4601:string)  [unwired: 2 in]
                                n1089 = Insert Into Array(array=w4602, index=5, new element=w4601) -> (w4599:string[])
                                }
                                n1090 = local write "loaded_lib"(w4592) -> ()
                                n1091 = local write "Librairie des objets"(w4593) -> ()
                                n1092 = local write "Librairie complète"(w4593) -> ()
                              }
                            }
                          }
                          frame True {
                          }
                        }
                      }
                      frame "scp_Charger la librairie Pesto" {
                        n1093 = local read "properties.ini"() -> (w4613:path)
                        n1094 = local read "path_libdir"() -> (w4616:path)
                        n1095 = call "Get_properties.vi"("Keyword"="pestolib" ("Section"), "Section"="chemins", "properties.ini"=w4613) -> ("error"=w4617:bool, "string"=w4615:string)  [unwired: 6 in, 1 out]
                        n1096 = case shown="Faux" w4617 {
                          tunnel: w4616 -> [w4625 _]
                          tunnel: w4615 -> [w4621 _]
                          tunnel: "table_technicien_pesto.dat" -> [w4631 _]
                          frame False {
                            n1097 = Build Path(base path=w4625, name or relative path=w4631) -> (appended path=w4630:path)
                            n1098 = File/Directory Info(path=w4630) -> (path out=w4627:path, error out=w4629:errorcluster)  [unwired: 1 in, 5 out]
                            n1099 = Unbundle By Name(w4629) -> ("status"=w4628:bool)
                            n1100 = local read "wgetexec"() -> (w4632:path)
                            n1101 = case shown="Faux" w4628 {
                              tunnel: w4627 -> [w4654 w4656]
                              tunnel: [w4653 w4656] -> w4626
                              tunnel: w4625 -> [w4652 w4655]
                              tunnel: [w4652 w4655] -> w4624
                              frame False {
                                n1102 = Delete(path (use dialog)=w4654) -> (deleted path=w4653:path)  [unwired: 4 in, 2 out]
                              }
                              frame True {
                              }
                            }
                            n1103 = Path To String(path=w4632) -> (string=w4622:string)
                            n1104 = Concatenate Strings(w4622, " " ("string"), w4621) -> (w4634:string)
                            n1105 = call <vilib>:"System Exec.vi"("run minimized? (F)"=TRUE, "working directory"=w4624, "command line"=w4634) -> ("error out"=w4623:errorcluster)  [unwired: 5 in, 3 out]
                            n1106 = flat-sequence {
                              tunnel: w4626 -> [w4638]
                              tunnel: w4623 -> [w4635]
                              frame #0 {
                                n1107 = local write "wget error"(w4635) -> ()
                                n1108 = call "Read_obs_files.vi"("Path"=w4638) -> ("path used"=w4636:path, "Output Table"=w4640:string[][])
                                n1109 = local read "LST"() -> (w4639:dbl)
                                n1110 = for {
                                tunnel: w4640 -> [w4646] mode=indexing
                                tunnel: w4639 -> [w4647]
                                tunnel: [w4643] -> w4637 mode=indexing
                                n1111 = Index Array(array=w4646, index #1=2 ("index"), index #2=3 ("index")) -> (element #1=w4649:string, element #2=w4648:string)
                                n1112 = call "Airmass.vi"("temps sidéral"=w4647, "DEC"=w4648, "RA"=w4649) -> ("airmass"=w4644:dbl)
                                n1113 = Number To Fractional String(number=w4644, precision (6)=i16 2) -> (F-format string=w4645:string)  [unwired: 2 in]
